vi "change control params.vi"(11 "PID exp exec in":T1={"T log file"={"log exists"=FALSE, "File refnum"=refnum, "temp log file path"=path ""}, "error"={"status"=FALSE, "code"=0, "source"=""}, "elapsed time (s)"=584.013}) -> (15 "PID exp exec in":T1={"T log file"={"log exists"=FALSE, "File refnum"=refnum, "temp log file path"=path ""}, "error"={"status"=FALSE, "code"=0, "source"=""}, "elapsed time (s)"=584.013})   [LabVIEW 2019]
doc: "Used as a popup subvi to allow the user to modify the current temperature control parameters.\n\nThe setpoint is part of the list for convenience, but not actionable. It's value is controlled by the executive setpoint instead; it is ovewrwritten is soon at the user finished editing the parameters and returns to execution via proceed.\n\nPaul K Dixon\nPhysics 350\nCSUSB Physics"
uses:
  typedefs/PID control parameters.ctl
  typedefs/PID exec cluster.ctl
  typedefs/bug temp file info.ctl
  globals/Bug temp globals.vi
panel:
  in  "Cancel Button":bool
  in  "OK Button":bool
  in  "Control Parameters":T3={"Setpoint"=30.0, "Control Bandwidth"=4.0, "Integral Time"=20.0, "Int\nON"=TRUE, "Derivative Tme"=0.4, "Der\nON"=TRUE, "Settle Bandwidth"=0.20000000000000007, "Settle Time"=60.0} {"Settle Time" step=1.0; "Settle Bandwidth" step=0.01; "Derivative Tme" step=0.01; "Integral Time" step=1.0; "Control Bandwidth" step=0.1; "Setpoint" step=0.1}
  # "Note:\nThe setpoint is controlled\nseperately\n\nthis instance is overwritten\nby the executive setpoint"
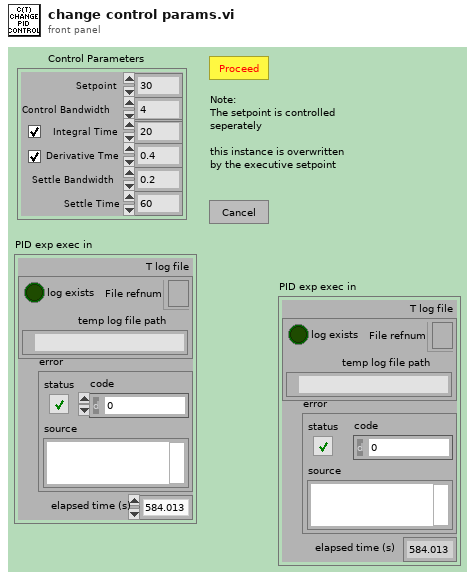
[diagram p1: front panel]
types:
  T1 = typedef "PID exec cluster.ctl" = cluster{"T log file":T2, "error":errorcluster, "elapsed time (s)":dbl}
  T2 = typedef "bug temp file info.ctl" = cluster{"log exists":bool, "File refnum":refnum<file>, "temp log file path":path}
  T3 = typedef "PID control parameters.ctl" = cluster{"Setpoint":dbl, "Control Bandwidth":dbl, "Integral Time":dbl, "Int\nON":bool, "Derivative Tme":dbl, "Der\nON":bool, "Settle Bandwidth":dbl, "Settle Time":dbl}
  T4 = typedef "temp cont cluster.ctl" = cluster{"exec":T5, "T status":T7, "T params":T3, "utility":T9}
  T5 = typedef "temp exec cluster.ctl" = cluster{"T mode":T6, "exec setpoint":dbl, "reset":bool, "man power":dbl, "man":bool, "log":bool, "clear":bool}
  T6 = typedef "temp mode enum.ctl" = enum16{"Setting up", "Listening to exec", "Exit"}
  T7 = typedef "temp indicator.ctl" = cluster{"Control status":T8, "Temp":dbl, "Power":dbl, "Time in settle band":dbl, "Settled":bool, "Low":bool, "High":bool, "Setpoint":dbl, "Control":bool, "In Settle Band":bool}
  T8 = typedef "temp control status.ctl" = enum16{"In Settle Band", "In Control Band", "Below Control Band", "Above Control Band"}
  T9 = typedef "temp cont utility.ctl" = cluster{"meas index":i32, "wait (ms)":i32, "H Vmax":dbl, "power out":dbl, "heat volt out":dbl, "heat volt in":dbl, "therm volt":dbl, "t T P hist":dbl[][], "cont hist":dbl[][]}
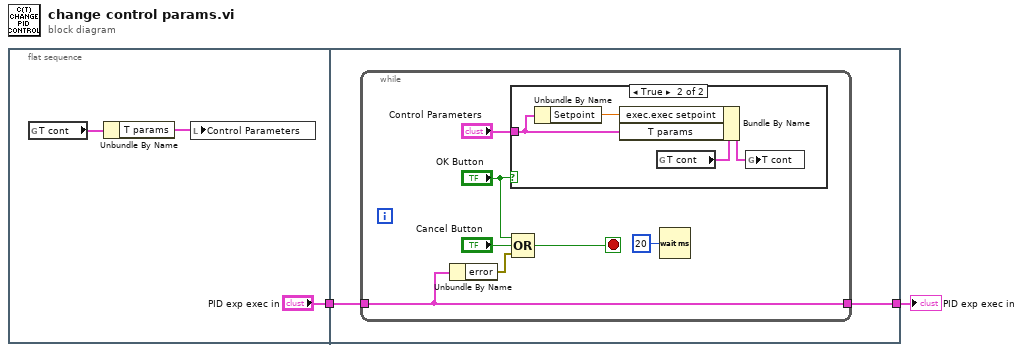
[diagram p0: block diagram]
diagram:
  n1 = flat-sequence {
    tunnel: ["PID exp exec in"] -> w2
    tunnel: w2 -> [w7]
    tunnel: [w6] -> w1
    frame #0 {
      n2 = global read "Bug temp globals.vi" "T cont"() -> (w5:T4)
      n3 = Unbundle By Name(w5) -> ("T params"=w4:T3)
      n4 = local write "Control Parameters"(w4) -> ()
    }
    frame #1 {
      n5 = while {
        tunnel: w7 -> [w9]
        tunnel: [w9] -> w6
        stop <- w14 stop-if-true
        n6 = Unbundle By Name(w9) -> ("error"=w8:errorcluster)
        n7 = case shown="True" "OK Button" {
          tunnel: "Control Parameters" -> [_ w16]
          frame False {
          }
          frame True {
            n8 = Unbundle By Name(w16) -> ("Setpoint"=w15:dbl)
            n9 = global read "Bug temp globals.vi" "T cont"() -> (w18:T4)
            n10 = Bundle By Name(cluster=w18, "exec.exec setpoint"=w15, "T params"=w16) -> (w17:T4)
            n11 = global write "Bug temp globals.vi" "T cont"(w17) -> ()
          }
        }
        n12 = Compound Arithmetic op=OR("OK Button", "Cancel Button", w8) -> (w14:bool)
        n13 = Wait (ms)(milliseconds to wait=u32 20) -> ()  [unwired: 1 out]
      }
    }
  }
  "PID exp exec in" <- w1
